vi "loadnilvce.vi"() -> ()   [LabVIEW 2020, in "XDNodeRunTimeDep.lvlib"]
uses:
  XDNodeRunTimeDep.lvlib
  nilvce.dll
panel:
  in  "Boolean":bool
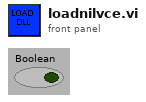
[diagram p1: front panel]
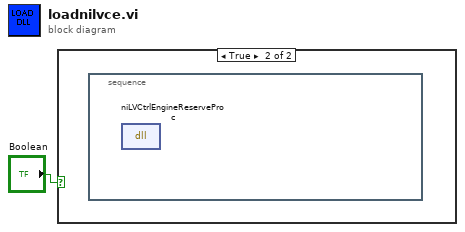
[diagram p0: block diagram]
diagram:
  n1 = case shown="True" "Boolean" {
    frame False {
    }
    frame True {
      n2 = stacked-sequence {
        frame #0 {
          n3 = dll-call lib="nilvce.*" fn="niLVCtrlEngineReserveProc" ("nilvce_wrapper.dll:niLVCtrlGetControllerState")() -> ()  [unwired: 4 in, 2 out]
        }
      }
    }
  }
